vi "CRYSet Option Setting Front Panel.vi"(11 "Vi Ref in":refnum<vi> caption="Vi Ref") -> (3 "Vi Ref out":refnum<vi> caption="Vi Ref")   [LabVIEW 2013]
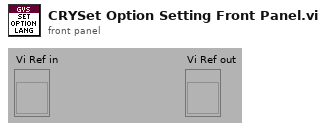
[diagram p1: front panel]
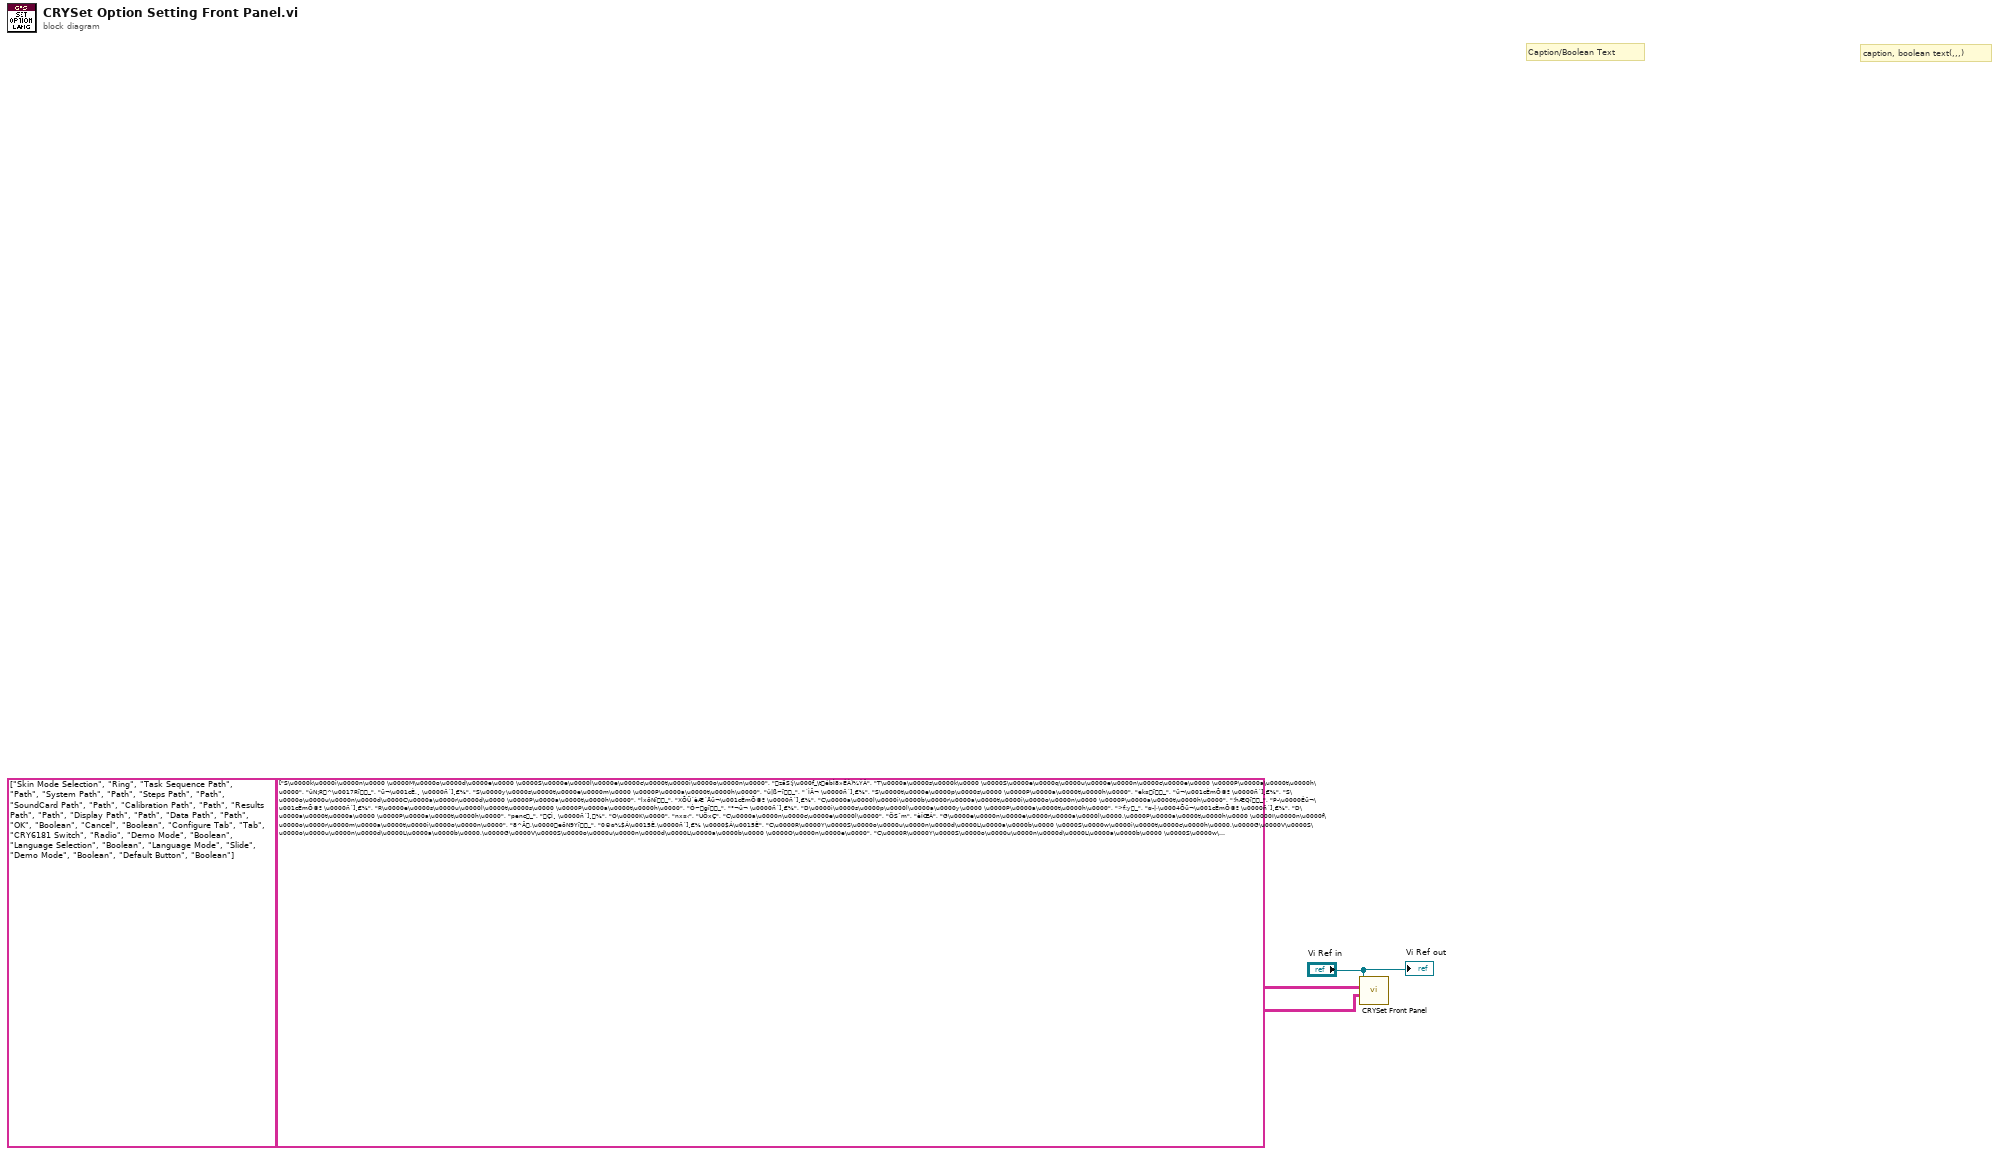
[diagram p0: block diagram]
diagram:
  # "caption, boolean text(,,,)"
  # "Caption/Boolean Text"
  n1 = call "CRYSet Front Panel.vi"("Caption(Boolean Text)"=string[][] [["S\u0000k\u0000i\u0000n\u0000 \u0000M\u0000o\u0000d\u0000e\u0000 \u0000S\u0000e\u0000l\u0000e\u0000c\u0000t\u0000i\u0000o\u0000n\u0000", "zãS!j\u000f_\téb", "=Ì8»ÉÀ)¼ÝÂ"], ["T\u0000a\u0000s\u0000k\u0000 \u0000S\u0000e\u0000q\u0000u\u0000e\u0000n\u0000c\u0000e\u0000 \u0000P\u0000a\u0000t\u0000h\u0000", "ûN¡R^\u0017Rï_", "ü¬\u001cÈ,¸ \u0000ñ´]¸€½"], ["S\u0000y\u0000s\u0000t\u0000e\u0000m\u0000 \u0000P\u0000a\u0000t\u0000h\u0000", "û|ß~ï_", "´ÌÄ¬ \u0000ñ´]¸€½"], ["S\u0000t\u0000e\u0000p\u0000s\u0000 \u0000P\u0000a\u0000t\u0000h\u0000", "ek¤ï_", "ü¬\u001cÈmÕ©º \u0000ñ´]¸€½"], ["S\u0000o\u0000u\u0000n\u0000d\u0000C\u0000a\u0000r\u0000d\u0000 \u0000P\u0000a\u0000t\u0000h\u0000", "lxöNï_", "XÕÜ´èÆ´Åü¬\u001cÈmÕ©º \u0000ñ´]¸€½"], ["C\u0000a\u0000l\u0000i\u0000b\u0000r\u0000a\u0000t\u0000i\u0000o\u0000n\u0000 \u0000P\u0000a\u0000t\u0000h\u0000", "!hÆQï_", "P­\u0000Éü¬\u001cÈmÕ©º \u0000ñ´]¸€½"], ["R\u0000e\u0000s\u0000u\u0000l\u0000t\u0000s\u0000 \u0000P\u0000a\u0000t\u0000h\u0000", "Ó~gï_", "°¬ü¬ \u0000ñ´]¸€½"], ["D\u0000i\u0000s\u0000p\u0000l\u0000a\u0000y\u0000 \u0000P\u0000a\u0000t\u0000h\u0000", ">f:y_", "ø­|·\u0004Õü¬\u001cÈmÕ©º \u0000ñ´]¸€½"], ["D\u0000a\u0000t\u0000a\u0000 \u0000P\u0000a\u0000t\u0000h\u0000", "penc_", "ÇÌ¸ \u0000ñ´]¸½"], ["O\u0000K\u0000", "nx¤‹", "UÖxÇ"], ["C\u0000a\u0000n\u0000c\u0000e\u0000l\u0000", "ÖSˆm", "èÍŒÁ"], ["G\u0000e\u0000n\u0000e\u0000r\u0000a\u0000l\u0000,\u0000P\u0000a\u0000t\u0000h\u0000 \u0000I\u0000n\u0000f\u0000o\u0000r\u0000m\u0000a\u0000t\u0000i\u0000o\u0000n\u0000", "8^Ä,\u0000eöN9Yï_", "0®ø¼$Á\u0015È,\u0000ñ´]¸€½ \u0000$Á\u0015È"], ["C\u0000R\u0000Y\u0000S\u0000o\u0000u\u0000n\u0000d\u0000L\u0000a\u0000b\u0000 \u0000S\u0000w\u0000i\u0000t\u0000c\u0000h\u0000,\u0000G\u0000V\u0000S\u0000o\u0000u\u0000n\u0000d\u0000L\u0000a\u0000b\u0000,\u0000G\u0000V\u0000S\u0000o\u0000u\u0000n\u0000d\u0000L\u0000a\u0000b\u0000 \u0000O\u0000n\u0000e\u0000", "C\u0000R\u0000Y\u0000S\u0000o\u0000u\u0000n\u0000d\u0000L\u0000a\u0000b\u0000 \u0000S\u0000w\u0000i\u0000t\u0000c\u0000h\u0000,\u0000¾|ðXðXf[ž[Œš¤[,\u0000¾|ðXðXf[ž[Œš¤[ \u0000\u0000N", "C\u0000R\u0000Y\u0000S\u0000o\u0000u\u0000n\u0000d\u0000L\u0000a\u0000b\u0000 \u0000S\u0000w\u0000i\u0000t\u0000c\u0000h\u0000,\u0000LÇ¥ÕtÕ\u001dÁ\u0004Õ\\¸ø­Œ·,\u0000LÇ¥ÕtÕ\u001dÁ\u0004Õ\\¸ø­Œ· \u0000XÕ˜°"], ["D\u0000e\u0000m\u0000o\u0000 \u0000M\u0000o\u0000d\u0000e\u0000", "\u0014o:y!j\u000f_", "ÜÂØÕ)¼ÝÂ"], ["L\u0000a\u0000n\u0000g\u0000u\u0000a\u0000g\u0000e\u0000 \u0000S\u0000e\u0000l\u0000e\u0000c\u0000t\u0000i\u0000o\u0000n\u0000", "í\u0000\téb", "¸Å´Å ÁÝÐ"], ["L\u0000a\u0000n\u0000g\u0000u\u0000a\u0000g\u0000e\u0000 \u0000M\u0000o\u0000d\u0000e\u0000,\u0000A\u0000u\u0000t\u0000o\u0000m\u0000a\u0000t\u0000i\u0000c\u0000,\u0000M\u0000a\u0000n\u0000u\u0000a\u0000l\u0000", "L\u0000a\u0000n\u0000g\u0000u\u0000a\u0000g\u0000e\u0000 \u0000M\u0000o\u0000d\u0000e\u0000,\u0000ê¨R,\u0000Kb¨R", "L\u0000a\u0000n\u0000g\u0000u\u0000a\u0000g\u0000e\u0000 \u0000M\u0000o\u0000d\u0000e\u0000,\u0000ÇÙ³,\u0000\u0018ÂÙ³"], ["T\u0000e\u0000s\u0000t\u0000 \u0000M\u0000o\u0000d\u0000e\u0000", "T\u0000e\u0000s\u0000t\u0000\u0000\u0000\u0000\u0000M\u0000o\u0000d\u0000e\u0000", "T\u0000e\u0000s\u0000t\u0000\u0000\u0000\u0000\u0000M\u0000o\u0000d\u0000e\u0000\u0000\u0000靛"], ["R\u0000e\u0000s\u0000t\u0000o\u0000r\u0000e\u0000 \u0000D\u0000e\u0000f\u0000a\u0000u\u0000l\u0000t\u0000", "b`\rYØž¤‹<P", "\\Ô\u0000É$Á\u0015È"]], "Control ID and Type(Label Name, Type)"=string[][] [["Skin Mode Selection", "Ring"], ["Task Sequence Path", "Path"], ["System Path", "Path"], ["Steps Path", "Path"], ["SoundCard Path", "Path"], ["Calibration Path", "Path"], ["Results Path", "Path"], ["Display Path", "Path"], ["Data Path", "Path"], ["OK", "Boolean"], ["Cancel", "Boolean"], ["Configure Tab", "Tab"], ["CRY6181 Switch", "Radio"], ["Demo Mode", "Boolean"], ["Language Selection", "Boolean"], ["Language Mode", "Slide"], ["Demo Mode", "Boolean"], ["Default Button", "Boolean"]], "Vi Ref"="Vi Ref in") -> ()  [unwired: 9 in]
  "Vi Ref out" <- "Vi Ref in"
